vi "Build Global Header.vi"(8 "error in (no error)":errorcluster, 9 "Override":u32=1, 10 "Link Types":T1, 11 "pcap Parse and Build in":refnum<class "pcap Parse and Build.lvclass">) -> (0 "error out":errorcluster, 2 "Global Header":u8[](array[numeric])=[161, 178, 60, 77, 0, 2, 0, 4, 0, 0, 0, 0, 0, 0, 0, 0, 0, 0, 255, 255, 0, 0, 0, 1] format="%.0x", 3 "pcap Parse and Build out":refnum<class "pcap Parse and Build.lvclass">)   [LabVIEW 2021, in "pcap Parse and Build.lvclass"]
uses:
  pcap Parse and Build.lvclass
  pcap Parse and Build.lvclass/pcap Parse and Build.ctl
  Typedef/Global Header.ctl
  Typedef/Link Types.ctl
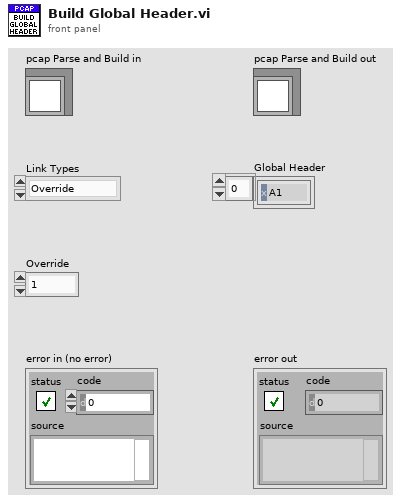
[diagram p1: front panel]
types:
  T1 = typedef "pcap Parse and Build.lvclass/Link Types.ctl" = enum16{"Override", "Ethernet", "Socket CAN", "I2C Linux"}
  T2 = typedef "pcap Parse and Build.lvclass/Global Header.ctl" = cluster{"magic number":u32, "Major Version":u16, "Minor Version":u16, "This Zone":u32, "Accuracy":u32, "Max Length":u32, "Data Link":u32}
  T3 = enum16{"big-endian, network order", "native, host order", "little-endian"}
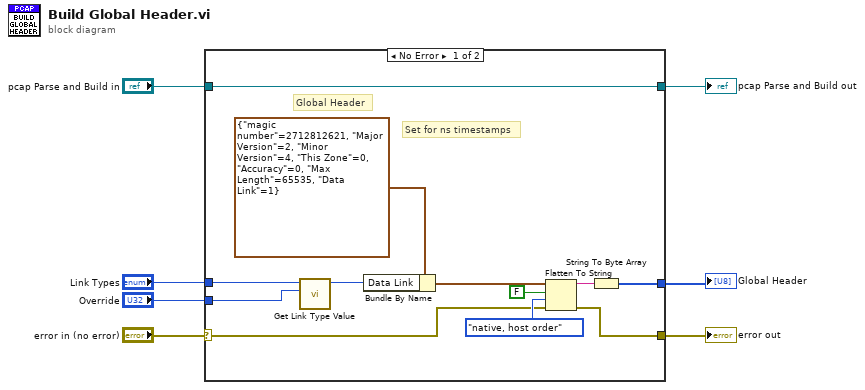
[diagram p0: block diagram]
diagram:
  n1 = case shown="No Error" "error in (no error)" {
    selector: "error in (no error)" -> [w10 w21]
    tunnel: [w9 w21] -> w6
    tunnel: [w19 w20] -> w4
    tunnel: "pcap Parse and Build in" -> [w19 w20]
    tunnel: "Override" -> [w13 _]
    tunnel: "Link Types" -> [w12 _]
    tunnel: [w8 _] -> w1
    frame No Error {
      # "Set for ns timestamps"
      # "Global Header"
      n2 = call "Get Link Type Value.vi"("Override"=w13, "Link Types"=w12) -> ("Link Type"=w14:u32)  [unwired: 9 in]
      n3 = Bundle By Name(cluster=T2 {"magic number"=2712812621, "Major Version"=2, "Minor Version"=4, "This Zone"=0, "Accuracy"=0, "Max Length"=65535, "Data Link"=1} ("Global Header"), "Data Link"=w14) -> (w15:T2)
      n4 = Flatten To String(anything=w15, prepend array or string size? (T)=FALSE, byte order (0:big-endian, network order)=T3."native, host order", error in (no error)=w10) -> (data string=w18:string, error out=w9:errorcluster)  [unwired: 1 out]
      n5 = String To Byte Array(string=w18) -> (unsigned byte array=w8:u8[])
    }
    frame Error {
    }
  }
  "error out" <- w6
  "pcap Parse and Build out" <- w4
  "Global Header" <- w1
